vi "Get Telemetry.vi"(8 "error in (no error)":errorcluster, 11 "S4ACS_GUI in":refnum<class "S4ACS_GUI.lvclass">) -> (0 "error out":errorcluster, 2 "TCS string":string, 3 "S4ACS_GUI out":refnum<class "S4ACS_GUI.lvclass">)   [LabVIEW 2018, in "S4ACS_GUI.lvclass"]
uses:
  S4ACS_GUI.lvclass
  S4ACS_GUI.lvclass/S4ACS_GUI.ctl
  TCS/TCS.lvclass
  Telemetry/Telemetry.lvclass
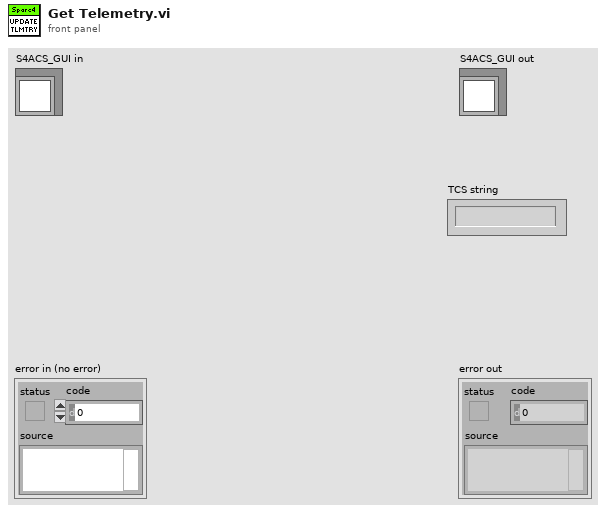
[diagram p1: front panel]
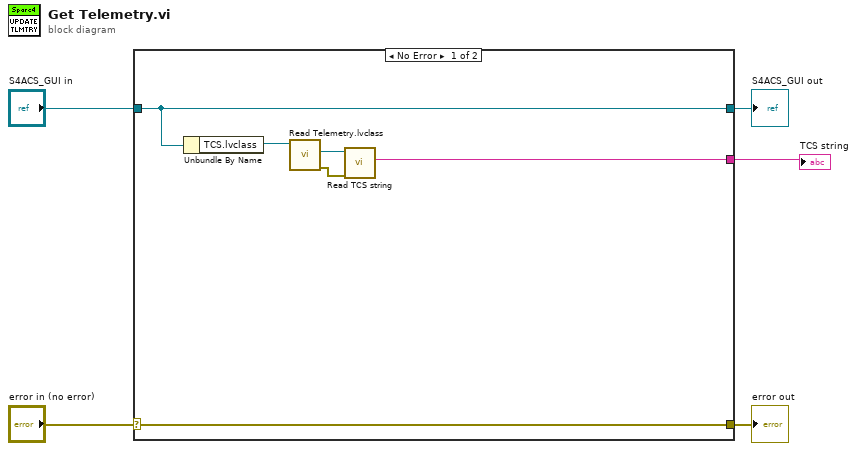
[diagram p0: block diagram]
diagram:
  n1 = case shown="No Error" "error in (no error)" {
    selector: "error in (no error)" -> [w6 w13]
    tunnel: [w6 w13] -> w4
    tunnel: [w7 w12] -> w2
    tunnel: "S4ACS_GUI in" -> [w7 w12]
    tunnel: [w8 _] -> w1
    frame No Error {
      n2 = Unbundle By Name(w7) -> ("TCS.lvclass"=w11:refnum<class "TCS.lvclass">)
      n3 = call-dynamic "Read Telemetry.lvclass.vi"("TCS in"=w11) -> ("error out"=w9:errorcluster, "Telemetry.lvclass"=w10:refnum<class "Telemetry.lvclass">)  [unwired: 8 in, 1 out]
      n4 = call-dynamic "Read TCS string.vi"("error in (no error)"=w9, "Telemetry in"=w10) -> ("TCS string"=w8:string)  [unwired: 7 in, 2 out]
    }
    frame Error {
    }
  }
  "error out" <- w4
  "S4ACS_GUI out" <- w2
  "TCS string" <- w1
